vi "thcd_chan_all.vi"(8 "err_in":errorcluster, 9 "thcd_b2r":u32, 10 "thcd_delay":u32=500, 11 "thcd_visa":refnum<visa-resource-name>) -> (3 "thcd_res":T2(array[cluster]), 4 "thcd_st":bool, 5 "thcd_res_str":string, 6 "err_out":errorcluster, 7 "thcd_visa":refnum<visa-resource-name>)   [LabVIEW 2020]
uses:
  mks946_controls/ctrl_chn_thcd.ctl
panel:
  out "thcd_res_4":T3
  out "thcd_res_3":T3
  out "thcd_res_2":T3
  out "thcd_res_1":T3
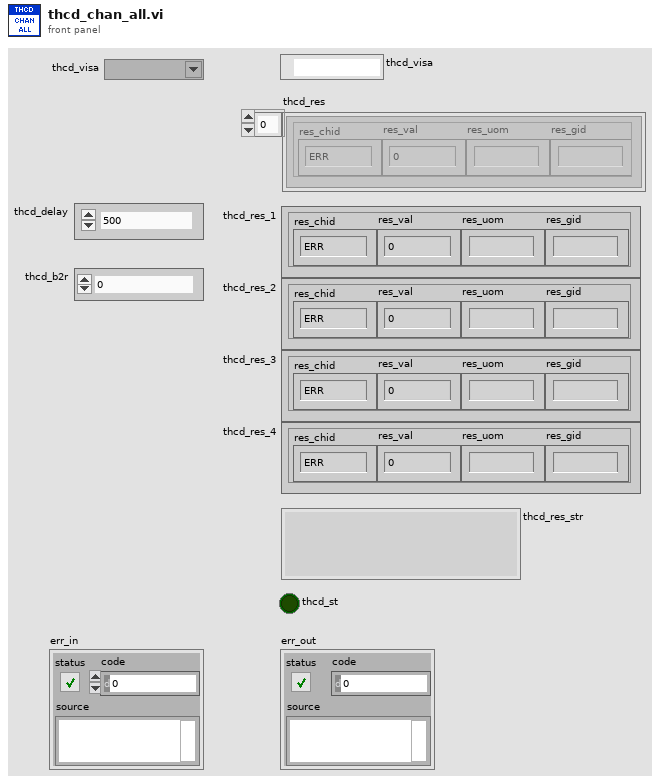
[diagram p1: front panel]
types:
  T1 = typedef "ctrl_chn_thcd.ctl" = enum8{"ERR", "1", "2", "3", "4"}
  T2 = cluster{"res_chid":T1, "res_val":dbl, "res_uom":string, "res_gid":string}[]
  T3 = cluster{"res_chid":T1, "res_val":dbl, "res_uom":string, "res_gid":string}
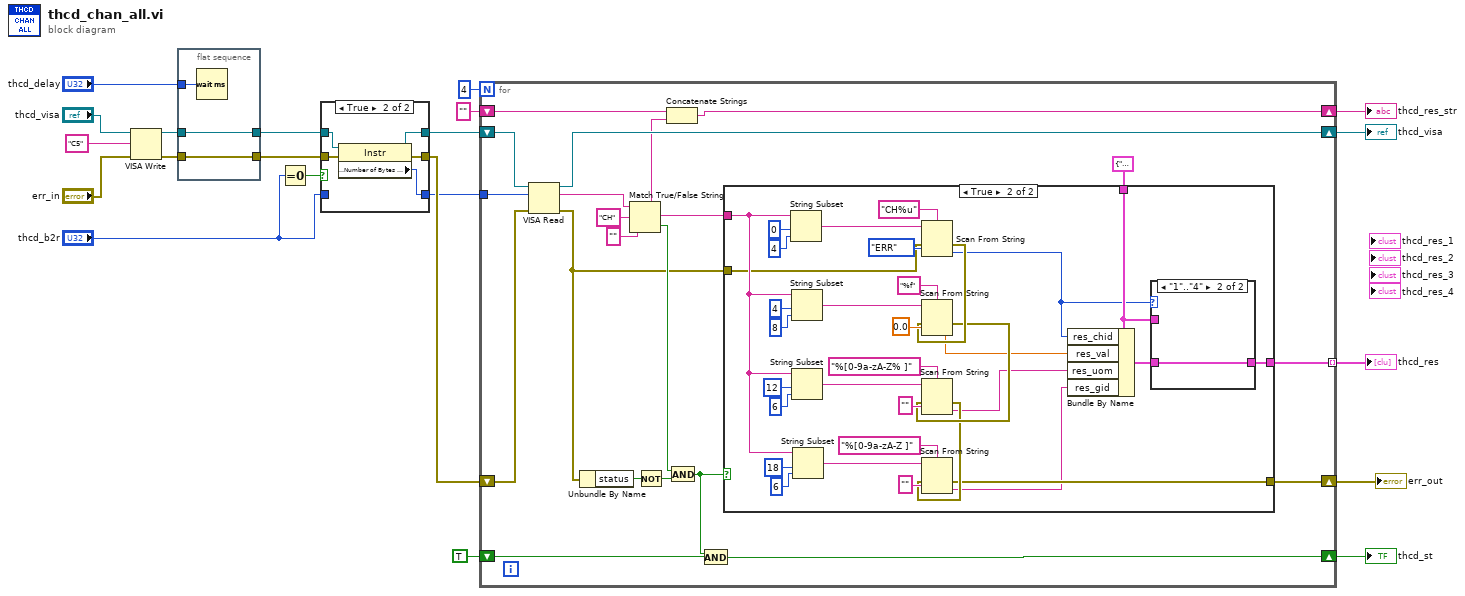
[diagram p0: block diagram]
diagram:
  n1 = VISA Write(VISA resource name="thcd_visa", write buffer="C5" ("format string"), error in (no error)="err_in") -> (VISA resource name out=w20:refnum<visa-resource-name>, error out=w21:errorcluster)  [unwired: 1 out]
  n2 = flat-sequence {
    tunnel: w21 -> [w23]
    tunnel: [w23] -> w14
    tunnel: w20 -> [w22]
    tunnel: [w22] -> w15
    tunnel: "thcd_delay" -> [w24]
    frame #0 {
      n3 = Wait (ms)(milliseconds to wait=w24) -> ()  [unwired: 1 out]
    }
  }
  n4 = Equal To 0?(x="thcd_b2r") -> (x = 0?=w16:bool)
  n5 = case shown="True" w16 {
    tunnel: [w26 w32] -> w13
    tunnel: [w25 w31] -> w12
    tunnel: [w27 w30] -> w11
    tunnel: "thcd_b2r" -> [w27 _]
    tunnel: w15 -> [w26 w29]
    tunnel: w14 -> [w25 w28]
    frame False {
    }
    frame True {
      n6 = property class="Instr"(reference=w29, error in=w28) -> (reference out=w32:refnum<visa-resource-name>, error out=w31:errorcluster, "Serial Settings:Number of Bytes at Serial Port"=w30:u32)
    }
  }
  n7 = for {
    N: 4 -> [_]
    tunnel: w11 -> [w49]
    shift-right: [w48] -> w8
    shift-left: w13 -> [w51]
    shift-right: [w33] -> w1
    shift-left: w12 -> [w50]
    tunnel: [w42] -> w6 mode=indexing
    shift-right: [w39] -> w2
    shift-left: "" -> [w40]
    shift-right: [w36] -> w3
    shift-left: TRUE -> [w37]
    n8 = VISA Read(VISA resource name=w51, byte count=w49, error in (no error)=w50) -> (VISA resource name out=w48:refnum<visa-resource-name>, read buffer=w38:string, error out=w34:errorcluster)  [unwired: 1 out]
    n9 = Unbundle By Name(w34) -> ("status"=w45:bool)
    n10 = Match True/False String(2:"" ("false string"), 3:"CH" ("true string"), 4:w38) -> (0:w44:bool)  [unwired: 1 out]
    n11 = Not(x=w45) -> (.not. x?=w43:bool)
    n12 = Concatenate Strings(w40, w38) -> (w39:string)
    n13 = And(x=w44, y=w43) -> (x .and. y?=w35:bool)
    n14 = And(x=w35, y=w37) -> (x .and. y?=w36:bool)
    n15 = case shown="True" w35 {
      tunnel: w38 -> [_ w75]
      tunnel: [w53 w86] -> w42
      tunnel: T3 {"res_chid"=enum."ERR", "res_val"=0.0, "res_uom"="", "res_gid"=""} ("res_1 2") -> [w53 w84]
      tunnel: w34 -> [w52 w62]
      tunnel: [w52 w58] -> w33
      frame False {
      }
      frame True {
        n16 = String Subset(string=w75, offset (0)=0, length (rest)=4 ("length (rest)")) -> (substring=w74:string)
        n17 = String Subset(string=w75, offset (0)=4, length (rest)=8 ("length (rest)")) -> (substring=w70:string)
        n18 = String Subset(string=w75, offset (0)=12, length (rest)=6 ("length (rest)")) -> (substring=w67:string)
        n19 = String Subset(string=w75, offset (0)=18, length (rest)=6 ("length (rest)")) -> (substring=w66:string)
        n20 = Scan From String(format string="CH%u", input string=w74, error in=w62, default 1=ctrl_chn_thcd."ERR" ("res_chid")) -> (error out=w61:errorcluster, output 1=w54:T1)  [unwired: 1 in, 2 out]
        n21 = Scan From String(format string="%f", input string=w70, error in=w61, default 1=0.0 ("default value 1")) -> (error out=w60:errorcluster, output 1=w57:dbl)  [unwired: 1 in, 2 out]
        n22 = Scan From String(format string="%[0-9a-zA-Z% ]", input string=w67, error in=w60, default 1="" ("default value 1")) -> (error out=w59:errorcluster, output 1=w56:string)  [unwired: 1 in, 2 out]
        n23 = Scan From String(format string="%[0-9a-zA-Z ]", input string=w66, error in=w59, default 1="" ("default value 1")) -> (error out=w58:errorcluster, output 1=w55:string)  [unwired: 1 in, 2 out]
        n24 = Bundle By Name(cluster=w84, "res_chid"=w54, "res_val"=w57, "res_uom"=w56, "res_gid"=w55) -> (w85:T3)
        n25 = case shown="\"1\"..\"4\"" w54 {
          tunnel: [w87 w88] -> w86
          tunnel: w85 -> [_ w88]
          tunnel: w84 -> [w87 _]
          frame "ERR", Default {
          }
          frame "1".."4" {
          }
        }
      }
    }
  }
  "err_out" <- w1
  "thcd_visa" <- w8
  "thcd_res_str" <- w2
  "thcd_st" <- w3
  "thcd_res" <- w6
